vi "initiation.vi"(2 "error in (no error)":errorcluster caption="错误输入（无错误）", 3 "StepMotor from file":refnum<class "StepMotor.lvclass">, 4 "StepMotor输入":refnum<class "StepMotor.lvclass">) -> (0 "error out":errorcluster caption="错误输出", 1 "StepMotor输出":refnum<class "StepMotor.lvclass">)   [LabVIEW 2016, in "MotionControl_UFO_3DOF.lvlib" / "StepMotor.lvclass"]
uses:
  <userlib>/MotionControl_UFO_3DOF/StepMotor/StepMotor.lvclass
  <userlib>/MotionControl_UFO_3DOF/StepMotor/StepMotor.lvclass/StepMotor.ctl
  <userlib>/UISimCanFunc_wrapper/UISimCanFunc_wrapper.lvlib
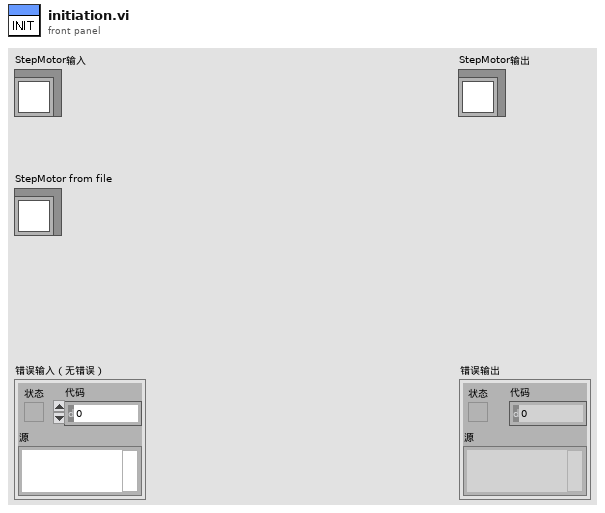
[diagram p1: front panel]
types:
  T1 = typedef "UISimCanFunc_wrapper.lvlib/UIM_MCFG_INFO_OBJ.ctl" = cluster{" bS1IE":bool, " bS2IE":bool, " bS3IE":bool, " bP4IE":bool, " bSTPIE":bool, " bORGIE":bool, " bSTLIE":bool, " bDM":bool, " bAM":bool, " bCM":bool, " bQEM":bool, " bQEI        ":bool, " bCHS":bool, " bANE":bool}
  T2 = typedef "UISimCanFunc_wrapper.lvlib/BASIC_ACK_OBJ.ctl" = cluster{"uiReserv":u32, "bENA":bool, "bDIR":bool, "bACR":bool, "uiMCS":u32, "uiCUR":u32, "uiSPD":u32, "uiSTP":u32}
  T3 = typedef "UISimCanFunc_wrapper.lvlib/MDL_INFO_OBJ.ctl" = cluster{"uiCANNodeType":u32, "uiCurrent":u32, "bIntegrationEncode":bool, "bEnCode":bool, "bMotion":bool, "b2Sensor":bool, "b4Sensor":bool, "uiFirewareVersion":u32, "szModelName":string}
  T4 = typedef "UISimCanFunc_wrapper.lvlib/UIM_ICFG_INFO_OBJ.ctl" = cluster{"bENA":bool, "bCCW":bool, "bPROG":bool, "bELOCK":bool, "bS1C":bool, "bS2C":bool, "bS3C":bool, "bP4C":bool}
  T5 = cluster{"uiS2RACT":u32, "uiS2FACT":u32, "uiS1RACT":u32, "uiS1FACT":u32}
  T6 = typedef "UISimCanFunc_wrapper.lvlib/DEV_INFO_OBJ.ctl" = cluster{"dwDevType":u32, "dwDevIndex":u32, " uiComIndex":u32, "uiBaudRate":u32, "pszDevName":string}
  T7 = typedef "UISimCanFunc_wrapper.lvlib/S34CON.ctl" = cluster{"bP4LVL":bool, "uiP4EVENT":u32, "uiS3RACT":u32, "uiS3FACT":u32, "uiSTLValue":u32}
  T8 = typedef "MotionControl_UFO_3DOF.lvlib/StepMotor.lvclass/AdvMovePara.ctl" = cluster{"acceleration":i32, "deceleration":i32, "max startup speed":i32, "max stop speed":i32}
  T9 = typedef "MotionControl_UFO_3DOF.lvlib/StepMotor.lvclass/UIM_ICFG.ctl" = cluster{"ENA-开机自动使能":bool, "CCW-设置电机正转向":bool, "UPG-上电自动执行用户程序":bool, "ELOCK-紧急上锁功能":bool, "S1C-开机使能S1":bool, "S2C-开机使能S2":bool, "S3C-开机使能S3":bool, "S4C-开机使能S4":bool}
  T10 = typedef "MotionControl_UFO_3DOF.lvlib/StepMotor.lvclass/UIM_MCFG.ctl" = cluster{"bS1IE":bool, "bS2IE":bool, "bS3IE":bool, "bP4IE":bool, "bSTPIE":bool, "bORGIE":bool, "bSTLIE":bool, "bDM":bool, "bAM":bool, "bCM":bool, "bQEM":bool, "bQEI":bool, "bCHS":bool, "bANE":bool}
  T11 = typedef "MotionControl_UFO_3DOF.lvlib/StepMotor.lvclass/S12CON.ctl" = cluster{"S2传感器上升沿绑定动作":u32, "S2传感器下降沿绑定动作":u32, "S1传感器上升沿绑定动作":u32, "S1传感器下降沿绑定动作":u32}
  T12 = typedef "MotionControl_UFO_3DOF.lvlib/StepMotor.lvclass/S34CON.ctl" = cluster{"TRUE: P4 出低电平; FALSE: P4 出高电平。":bool, "P4输出关联的事件代码":u32, "S3传感器上升沿绑定动作":u32, "S3传感器下降沿绑定动作":u32, "当发生堵转时动作":u32}
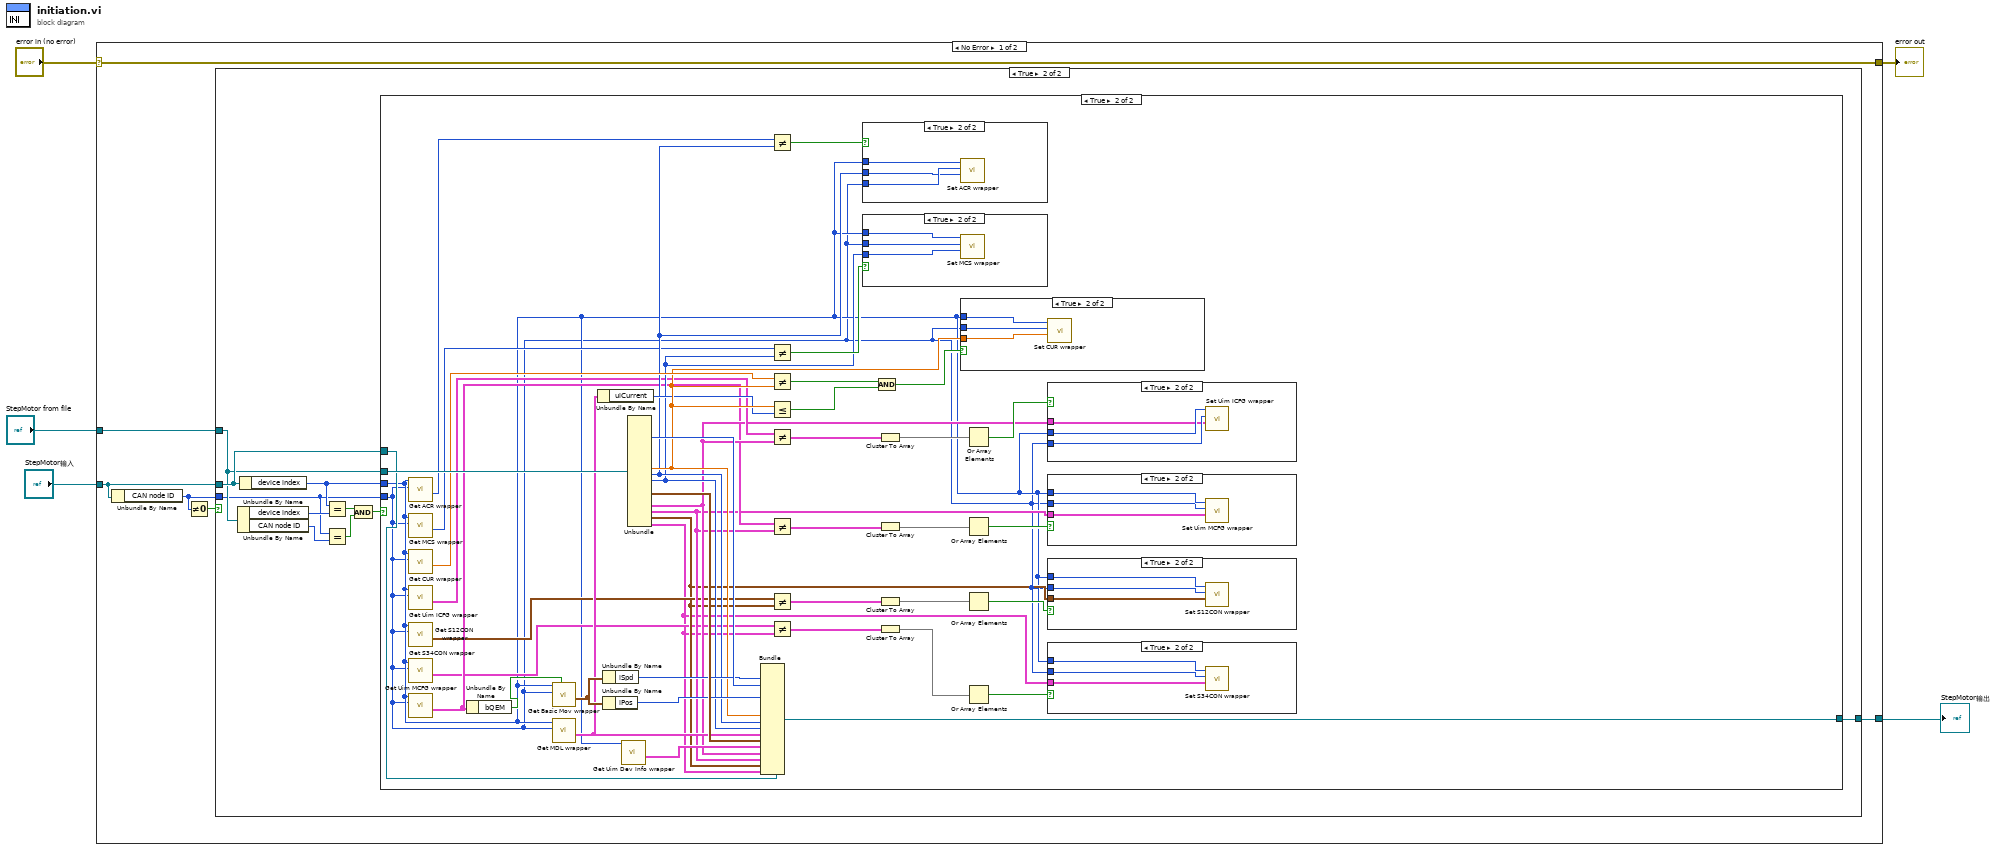
[diagram p0: block diagram]
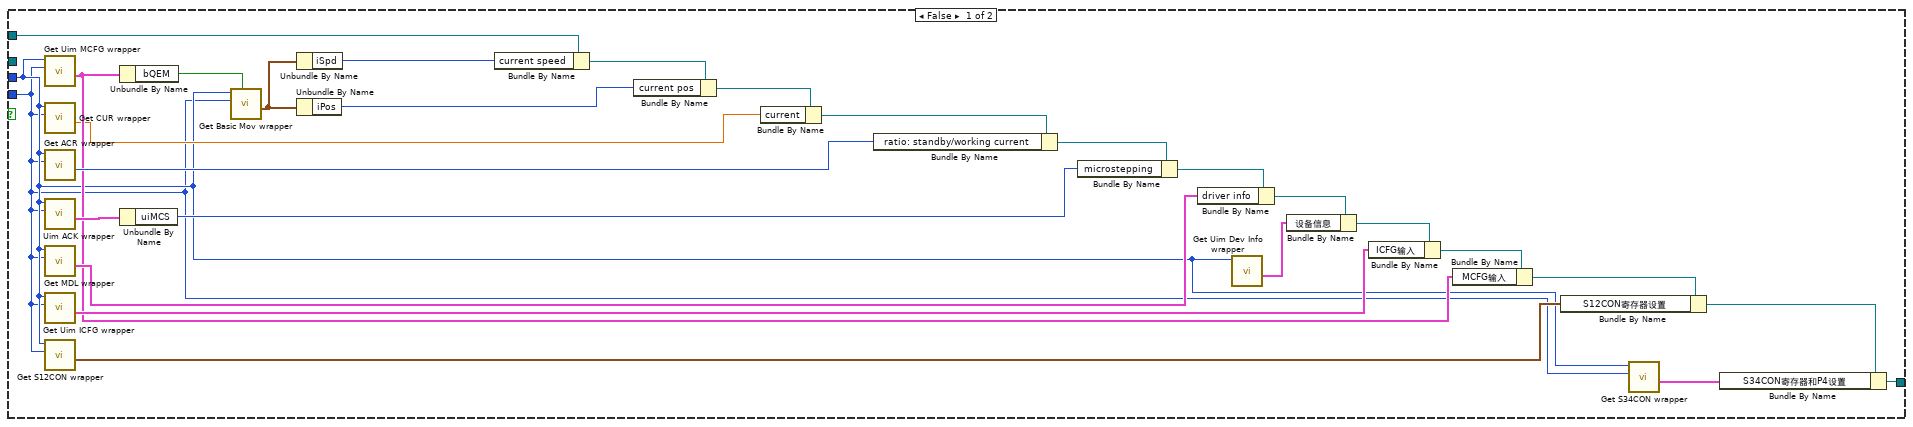
[diagram p3: hidden frame]
diagram:
  n1 = case shown="No Error" "error in (no error)" {
    selector: "error in (no error)" -> [w11 w118]
    tunnel: [w11 w118] -> w4
    tunnel: [w10 w117] -> w2
    tunnel: "StepMotor输入" -> [w8 w117]
    tunnel: "StepMotor from file" -> [w9 _]
    frame No Error {
      n2 = Unbundle By Name(w8) -> ("CAN node ID"=w7:u32)
      n3 = Not Equal To 0?(x=w7) -> (x != 0?=w6:bool)
      n4 = case shown="True" w6 {
        tunnel: w8 -> [w12 w22]
        tunnel: [w12 w21] -> w10
        tunnel: w9 -> [_ w15]
        tunnel: w7 -> [_ w14]
        frame False {
        }
        frame True {
          n5 = Unbundle By Name(w15) -> ("device index"=w19:u32, "CAN node ID"=w13:u32)
          n6 = Unbundle By Name(w22) -> ("device index"=w20:u32)
          n7 = Equal?(x=w20, y=w19) -> (x = y?=w18:bool)
          n8 = Equal?(x=w14, y=w13) -> (x = y?=w17:bool)
          n9 = Compound Arithmetic op=AND(w18, w17) -> (w16:bool)
          n10 = case shown="True" w16 {
            tunnel: w22 -> [w47 w94]
            tunnel: [w28 w51] -> w21
            tunnel: w20 -> [w24 w54]
            tunnel: w14 -> [w23 w53]
            tunnel: w15 -> [_ w95]
            frame False {
              n11 = call <userlib>:"Get Uim MCFG wrapper.vi"("dwCanNodeId"=w23, "dwDevIndex"=w24) -> ("UIM_MCFG_INFO_OBJ"=w31:T1)  [unwired: 7 in, 2 out]
              n12 = call <userlib>:"Get CUR wrapper.vi"("dwCanNodeId"=w23, "dwDevIndex"=w24) -> ("current"=w25:dbl)  [unwired: 7 in, 2 out]
              n13 = call <userlib>:"Get ACR wrapper.vi"("dwCanNodeId"=w23, "dwDevIndex"=w24) -> ("pRtnValue out"=w43:i32)  [unwired: 7 in, 2 out]
              n14 = call <userlib>:"Uim ACK wrapper.vi"("dwCanNodeId"=w23, "dwDevIndex"=w24) -> ("BASIC_ACK_OBJ"=w50:T2)  [unwired: 7 in, 2 out]
              n15 = call <userlib>:"Get MDL wrapper.vi"("dwCanNodeId"=w23, "dwDevIndex"=w24) -> ("MDL_INFO_OBJ"=w38:T3)  [unwired: 7 in, 2 out]
              n16 = call <userlib>:"Get Uim ICFG wrapper.vi"("dwCanNodeId"=w23, "dwDevIndex"=w24) -> ("UIM_ICFG_INFO_OBJ"=w32:T4)  [unwired: 7 in, 2 out]
              n17 = call <userlib>:"Get S12CON wrapper.vi"("dwCanNodeId"=w23, "dwDevIndex"=w24) -> ("pS12Con out"=w30:T5)  [unwired: 7 in, 2 out]
              n18 = Unbundle By Name(w31) -> ("bQEM"=w48:bool)
              n19 = Unbundle By Name(w50) -> ("uiMCS"=w41:u32)
              n20 = call <userlib>:"Get Basic Mov wrapper.vi"("bLoop"=w48, "dwCanNodeId"=w23, "dwDevIndex"=w24) -> ("pBasicMovObj out"=w49:cluster{"iSpd":i32, "iPos":i32, "iTimeOut":i32})  [unwired: 6 in, 2 out]
              n21 = Unbundle By Name(w49) -> ("iSpd"=w46:i32)
              n22 = Unbundle By Name(w49) -> ("iPos"=w44:i32)
              n23 = Bundle By Name(cluster=w47, "current speed"=w46) -> (w45:refnum<class "StepMotor.lvclass">)
              n24 = Bundle By Name(cluster=w45, "current pos"=w44) -> (w27:refnum<class "StepMotor.lvclass">)
              n25 = Bundle By Name(cluster=w27, "current"=w25) -> (w26:refnum<class "StepMotor.lvclass">)
              n26 = Bundle By Name(cluster=w26, "ratio: standby/working current"=w43) -> (w42:refnum<class "StepMotor.lvclass">)
              n27 = Bundle By Name(cluster=w42, "microstepping"=w41) -> (w40:refnum<class "StepMotor.lvclass">)
              n28 = Bundle By Name(cluster=w40, "driver info"=w38) -> (w39:refnum<class "StepMotor.lvclass">)
              n29 = call <userlib>:"Get Uim Dev Info wrapper.vi"("dwDevIndex"=w24) -> ("DEV_INFO_OBJ"=w37:T6)  [unwired: 8 in, 2 out]
              n30 = Bundle By Name(cluster=w39, "设备信息"=w37) -> (w36:refnum<class "StepMotor.lvclass">)
              n31 = Bundle By Name(cluster=w36, "ICFG输入"=w32) -> (w35:refnum<class "StepMotor.lvclass">)
              n32 = Bundle By Name(cluster=w35, "MCFG输入"=w31) -> (w34:refnum<class "StepMotor.lvclass">)
              n33 = Bundle By Name(cluster=w34, "S12CON寄存器设置"=w30) -> (w33:refnum<class "StepMotor.lvclass">)
              n34 = call <userlib>:"Get S34CON wrapper.vi"("dwCanNodeId"=w23, "dwDevIndex"=w24) -> ("S34CON"=w29:T7)  [unwired: 7 in, 2 out]
              n35 = Bundle By Name(cluster=w33, "S34CON寄存器和P4设置"=w29) -> (w28:refnum<class "StepMotor.lvclass">)
            }
            frame True {
              n36 = call <userlib>:"Get ACR wrapper.vi"("dwCanNodeId"=w53, "dwDevIndex"=w54) -> ("pRtnValue out"=w79:i32)  [unwired: 7 in, 2 out]
              n37 = call <userlib>:"Get MCS wrapper.vi"("dwCanNodeId"=w53, "dwDevIndex"=w54) -> ("MCS"=w74:i32)  [unwired: 7 in, 2 out]
              n38 = call <userlib>:"Get CUR wrapper.vi"("dwCanNodeId"=w53, "dwDevIndex"=w54) -> ("current"=w86:dbl)  [unwired: 7 in, 2 out]
              n39 = call <userlib>:"Get Uim ICFG wrapper.vi"("dwCanNodeId"=w53, "dwDevIndex"=w54) -> ("UIM_ICFG_INFO_OBJ"=w73:T4)  [unwired: 7 in, 2 out]
              n40 = call <userlib>:"Get S12CON wrapper.vi"("dwCanNodeId"=w53, "dwDevIndex"=w54) -> ("pS12Con out"=w57:T5)  [unwired: 7 in, 2 out]
              n41 = call <userlib>:"Get S34CON wrapper.vi"("dwCanNodeId"=w53, "dwDevIndex"=w54) -> ("S34CON"=w55:T7)  [unwired: 7 in, 2 out]
              n42 = call <userlib>:"Get Uim MCFG wrapper.vi"("dwCanNodeId"=w53, "dwDevIndex"=w54) -> ("UIM_MCFG_INFO_OBJ"=w59:T1)  [unwired: 7 in, 2 out]
              n43 = Unbundle By Name(w59) -> ("bQEM"=w90:bool)
              n44 = call <userlib>:"Get Basic Mov wrapper.vi"("bLoop"=w90, "dwCanNodeId"=w53, "dwDevIndex"=w54) -> ("pBasicMovObj out"=w91:cluster{"iSpd":i32, "iPos":i32, "iTimeOut":i32})  [unwired: 6 in, 2 out]
              n45 = call <userlib>:"Get MDL wrapper.vi"("dwCanNodeId"=w53, "dwDevIndex"=w54) -> ("MDL_INFO_OBJ"=w85:T3)  [unwired: 7 in, 2 out]
              n46 = Unbundle By Name(w85) -> ("uiCurrent"=w83:u32)
              n47 = Unbundle By Name(w91) -> ("iSpd"=w89:i32)
              n48 = Unbundle By Name(w91) -> ("iPos"=w88:i32)
              n49 = call <userlib>:"Get Uim Dev Info wrapper.vi"("dwDevIndex"=w54) -> ("DEV_INFO_OBJ"=w87:T6)  [unwired: 8 in, 2 out]
              n50 = Unbundle(w95) -> (w93:i32, w84:dbl, w76:i32, w75:u32, w92:T8, w60:T9, w58:T10, w56:T11, w52:T12)  [unwired: 9 out]
              n51 = Bundle(cluster=w94, w89, w93, w88, w84, w76, w75, w85, w92, w87, w60, w58, w56, w52) -> (w51:refnum<class "StepMotor.lvclass">)  [unwired: 5 in]
              n52 = Not Equal?(x=w79, y=w76) -> (x != y?=w78:bool)
              n53 = Not Equal?(x=w74, y=w75) -> (x != y?=w77:bool)
              n54 = Not Equal?(x=w86, y=w84) -> (x != y?=w81:bool)
              n55 = Less Or Equal?(x=w84, y=w83) -> (x <= y?=w82:bool)
              n56 = Not Equal?(x=w73, y=w60) -> (x != y?=w72:T4)
              n57 = Not Equal?(x=w59, y=w58) -> (x != y?=w69:T1)
              n58 = Not Equal?(x=w57, y=w56) -> (x != y?=w66:cluster{bool, bool, bool, bool})
              n59 = Not Equal?(x=w55, y=w52) -> (x != y?=w63:cluster{bool, bool, bool, bool, bool})
              n60 = case shown="True" w78 {
                tunnel: w54 -> [_ w113]
                tunnel: w53 -> [_ w112]
                tunnel: w76 -> [_ w111]
                frame False {
                }
                frame True {
                  n61 = call <userlib>:"Set ACR wrapper.vi"("iACR"=w111, "dwCanNodeId"=w112, "dwDevIndex"=w113) -> ()  [unwired: 6 in, 3 out]
                }
              }
              n62 = case shown="True" w77 {
                tunnel: w54 -> [_ w110]
                tunnel: w53 -> [_ w109]
                tunnel: w75 -> [_ w108]
                frame False {
                }
                frame True {
                  n63 = call <userlib>:"Set MCS wrapper.vi"("iMCS"=w108, "dwCanNodeId"=w109, "dwDevIndex"=w110) -> ()  [unwired: 6 in, 3 out]
                }
              }
              n64 = And(x=w81, y=w82) -> (x .and. y?=w80:bool)
              n65 = Cluster To Array(cluster=w72) -> (array=w71:bool[])
              n66 = Cluster To Array(cluster=w69) -> (array=w68:bool[])
              n67 = Cluster To Array(cluster=w66) -> (array=w65:bool[])
              n68 = Cluster To Array(cluster=w63) -> (array=w62:bool[])
              n69 = case shown="True" w80 {
                tunnel: w54 -> [_ w116]
                tunnel: w53 -> [_ w115]
                tunnel: w84 -> [_ w114]
                frame False {
                }
                frame True {
                  n70 = call <userlib>:"Set CUR wrapper.vi"("fCUR"=w114, "dwCanNodeId"=w115, "dwDevIndex"=w116) -> ()  [unwired: 6 in, 3 out]
                }
              }
              n71 = Or Array Elements(Boolean array=w71) -> (logical OR=w70:bool)
              n72 = Or Array Elements(Boolean array=w68) -> (logical OR=w67:bool)
              n73 = Or Array Elements(Boolean array=w65) -> (logical OR=w64:bool)
              n74 = Or Array Elements(Boolean array=w62) -> (logical OR=w61:bool)
              n75 = case shown="True" w70 {
                tunnel: w54 -> [_ w107]
                tunnel: w53 -> [_ w106]
                tunnel: w60 -> [_ w105]
                frame False {
                }
                frame True {
                  n76 = call <userlib>:"Set Uim ICFG wrapper.vi"("UIM_ICFG_INFO_OBJ In"=w105, "dwCanNodeId"=w106, "dwDevIndex"=w107) -> ()  [unwired: 6 in, 3 out]
                }
              }
              n77 = case shown="True" w67 {
                tunnel: w54 -> [_ w104]
                tunnel: w53 -> [_ w103]
                tunnel: w58 -> [_ w102]
                frame False {
                }
                frame True {
                  n78 = call <userlib>:"Set Uim MCFG wrapper.vi"("UIM_MCFG_INFO_OBJ In"=w102, "dwCanNodeId"=w103, "dwDevIndex"=w104) -> ()  [unwired: 6 in, 3 out]
                }
              }
              n79 = case shown="True" w64 {
                tunnel: w54 -> [_ w101]
                tunnel: w53 -> [_ w100]
                tunnel: w56 -> [_ w99]
                frame False {
                }
                frame True {
                  n80 = call <userlib>:"Set S12CON wrapper.vi"("pS12ConIn"=w99, "dwCanNodeId"=w100, "dwDevIndex"=w101) -> ()  [unwired: 6 in, 3 out]
                }
              }
              n81 = case shown="True" w61 {
                tunnel: w54 -> [_ w98]
                tunnel: w53 -> [_ w97]
                tunnel: w52 -> [_ w96]
                frame False {
                }
                frame True {
                  n82 = call <userlib>:"Set S34CON wrapper.vi"("S34CON In"=w96, "dwCanNodeId"=w97, "dwDevIndex"=w98) -> ()  [unwired: 6 in, 3 out]
                }
              }
            }
          }
        }
      }
    }
    frame Error {
    }
  }
  "error out" <- w4
  "StepMotor输出" <- w2
